vi "Write Return FIFO.vi"(8 "error in (no error)":errorcluster, 9 "timeout in ms (0)":i32 format="%d ms", 11 "Transfer Group in":refnum<class "Transfer Group.lvclass">) -> (0 "error out":errorcluster, 1 "timed out?":bool, 3 "Transfer Group out":refnum<class "Transfer Group.lvclass">)   [LabVIEW 2019, in "DSF Core.lvlib" / "Transfer Group.lvclass"]
uses:
  Transfer Group.lvclass
  Transfer Group.lvclass/Transfer Group.ctl
  Timing/Timing.lvclass
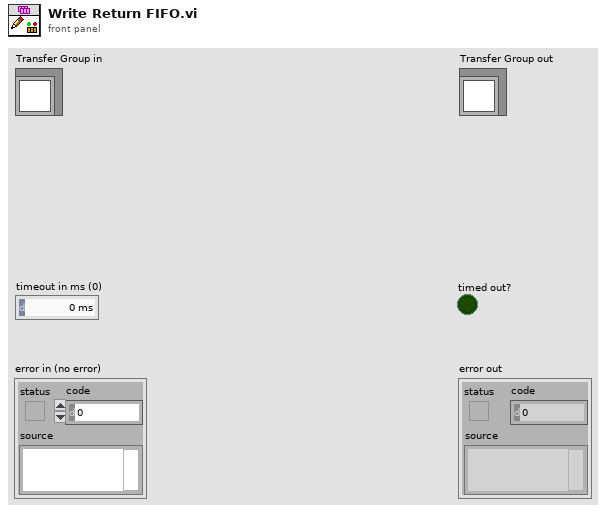
[diagram p1: front panel]
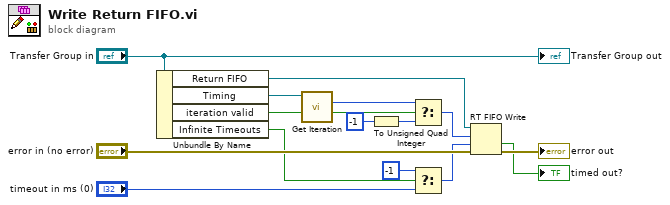
[diagram p0: block diagram]
diagram:
  n1 = Unbundle By Name("Transfer Group in") -> ("Return FIFO"=w9:refnum<k33>, "Timing"=w7:refnum<class "Timing.lvclass">, "iteration valid"=w2:bool, "Infinite Timeouts"=w1:bool)
  n2 = call "Get Iteration.vi"("Timing in"=w7) -> ("Iteration"=w6:u64)  [unwired: 9 in, 1 out]
  n3 = To Unsigned Quad Integer(1:i64 -1) -> (0:w3:u64)
  n4 = Select(t=w6, s=w2, f=w3) -> (s? t:f=w5:u64)
  n5 = Select(t=-1, s=w1, f="timeout in ms (0)") -> (s? t:f=w10:i32)
  n6 = RT FIFO Write(0:w9, 1:w5, 2:w10, 3:"error in (no error)") -> (10:→"timed out?":bool, 11:→"error out":errorcluster)  [unwired: 1 in, 2 out]
  "Transfer Group out" <- "Transfer Group in"
